vi "SubMatrix.vi"() -> ()   [LabVIEW 2014]
uses:
  <vilib>/Utility/file.llb/Read From Spreadsheet File (I64).vi
panel:
  in  "From V2 to 0":bool caption="From 0 to V1"
  in  "GPIB":string="12"
  in  "Sweep Rate w/o recording (V/min)":dbl=30.0
  in  "From V1 to V2":bool=TRUE
  in  "From 0 to V1":bool
  in  "Sweep Rate (V/min)":dbl=0.6
  in  "Menu Ring":u16(ring) caption="Show configuration:" items=["Configuration #1", "Configuration #2", "Configuration #3"]
  in  "Start Sweep":bool
  out "# of configurations":dbl
  out "Configuration file:":path
  in  "V2 (V)":dbl=2.1
  in  "V1 (V)":dbl=-2.1
  out "Array":bool[][](array[boolean])
  # "Which part of sweep to be recorded?"
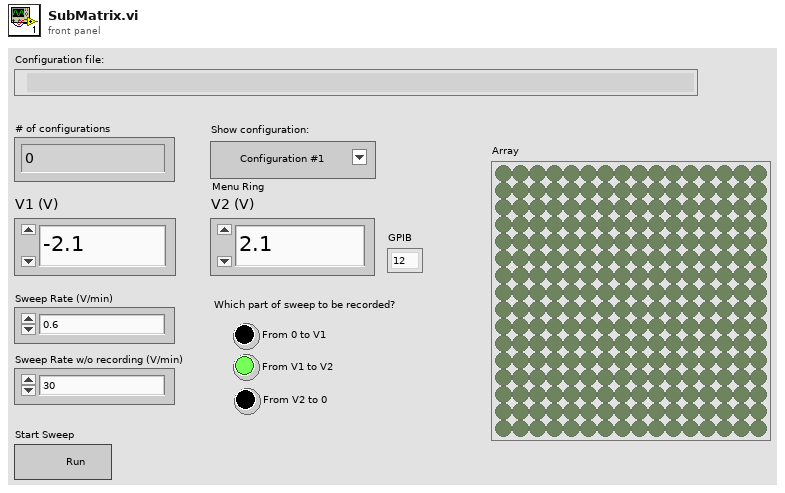
[diagram p1: front panel]
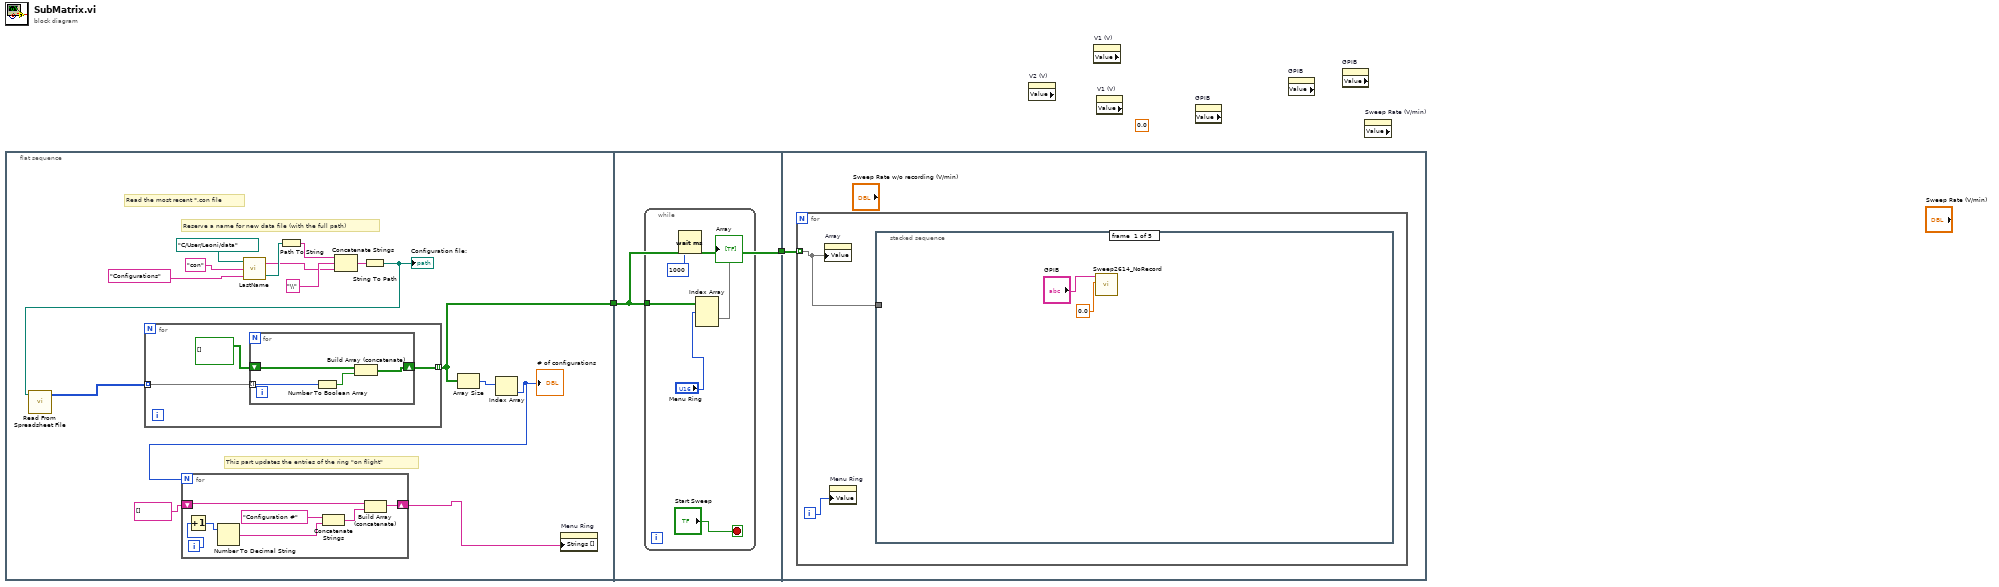
[diagram p0: block diagram]
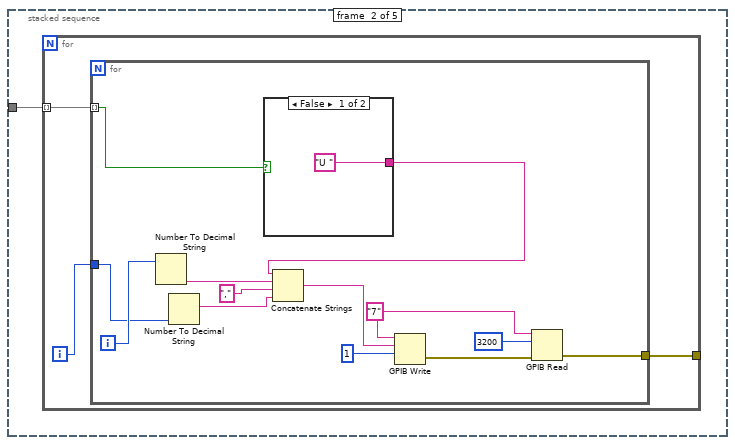
[diagram p2: hidden frame]
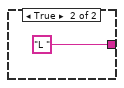
[diagram p3: hidden frame]
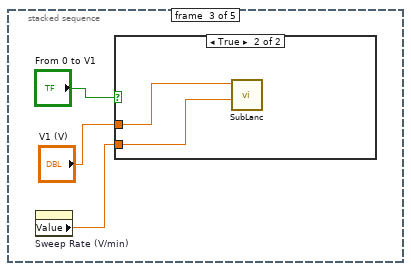
[diagram p4: hidden frame]
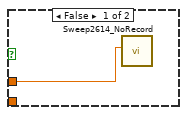
[diagram p5: hidden frame]
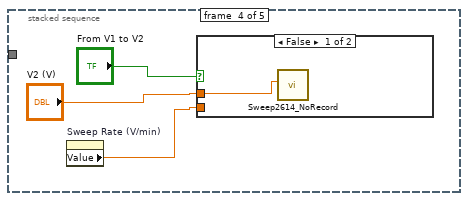
[diagram p6: hidden frame]
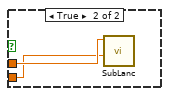
[diagram p7: hidden frame]
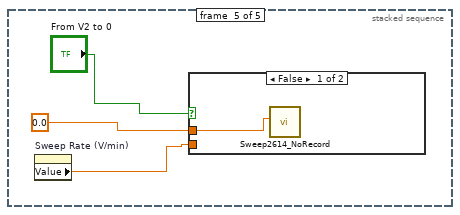
[diagram p8: hidden frame]
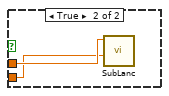
[diagram p9: hidden frame]
diagram:
  (unwired) 0.0
  n1 = flat-sequence {
    tunnel: [w4] -> w2
    tunnel: w2 -> [w32]
    tunnel: [w32] -> w1
    tunnel: w1 -> [w38]
    frame #0 {
      # "This part updates the entries of the ring \"on flight\""
      # "Reserve a name for new data file (with the full path)"
      # "Read the most recent *.con file"
      n2 = call "LastName.vi"("Custom Folder"="Configurations", "Extention"="con", "User Data Folder"=path "C:/User/Leoni/data") -> ("created path"=w13:path, "String"=w12:string)
      n3 = Path To String(path=w13) -> (string=w17:string)
      n4 = Concatenate Strings(w17, "\\", w12) -> (w15:string)
      n5 = String To Path(string=w15) -> (path=w9:path)
      "Configuration file:" <- w9
      n6 = call-poly <vilib>:"Read From Spreadsheet File.vi"("file path (dialog if empty)"=w9) -> ("all rows"=w8:i64[][])  [unwired: 6 in, 4 out]
      n7 = for {
        tunnel: w8 -> [w27] mode=indexing
        tunnel: [w26] -> w4 mode=indexing
        n8 = for {
          tunnel: w27 -> [w31] mode=indexing
          shift-right: [w28] -> w26
          shift-left: bool[][] [] -> [w29]
          n9 = Number To Boolean Array(number=w31) -> (Boolean array=w30:bool[])
          n10 = Build Array (concatenate)(w29, w30) -> (w28:bool[][])
        }
      }
      n11 = Array Size(array=w4) -> (size(s)=w7:i32[])
      n12 = Index Array(array=w7) -> (element=w5:i32)  [unwired: 1 in]
      "# of configurations" <- w5
      n13 = for {
        N: w5 -> [_]
        shift-right: [w21] -> w3
        shift-left: string[] [] -> [w22]
        i -> [w19]
        n14 = Increment(x=w19) -> (x+1=w18:i32)
        n15 = Number To Decimal String(number=w18) -> (decimal integer string=w23:string)  [unwired: 1 in]
        n16 = Concatenate Strings("Configuration #", w23) -> (w20:string)
        n17 = Build Array (concatenate)(w22, w20) -> (w21:string[])
      }
      n18 = property on="Menu Ring" class="Ring (strict)"("Strings []"=w3) -> ()  [unwired: 2 in, 2 out]
    }
    frame #1 {
      n19 = while {
        tunnel: w32 -> [w37]
        stop <- "Start Sweep" stop-if-true
        n20 = Wait (ms)(milliseconds to wait=1000) -> ()  [unwired: 1 out]
        n21 = Index Array(array=w37, index (dim 0)="Menu Ring") -> (element=→"Array":bool[][])  [unwired: 2 in]
      }
    }
    frame #2 {
      n22 = for {
        tunnel: w38 -> [w39] mode=indexing
        i -> [w40]
        n23 = property on="Array" class="Arr (strict)"("Value"=w39) -> ()  [unwired: 2 in, 2 out]
        n24 = property on="Menu Ring" class="Ring (strict)"("Value"=w40) -> ()  [unwired: 2 in, 2 out]
        n25 = stacked-sequence {
          tunnel: w39 -> [_ w43 _ _ _]
          frame #0 {
            n26 = call "Sweep2614_NoRecord.vi"("Vfinal (V)"=0.0, "GPIB"="GPIB") -> ()  [unwired: 2 in, 1 out]
          }
          frame #1 {
            n27 = for {
              tunnel: [w45] -> _
              tunnel: w43 -> [w44] mode=indexing
              i -> [w46]
              n28 = for {
                tunnel: w46 -> [w48]
                tunnel: [w51] -> w45
                tunnel: w44 -> [w47] mode=indexing
                i -> [w49]
                w53 = "7"
                n29 = Number To Decimal String(number=w49) -> (decimal integer string=w58:string)  [unwired: 1 in]
                n30 = Number To Decimal String(number=w48) -> (decimal integer string=w57:string)  [unwired: 1 in]
                n31 = case shown="False" w47 {
                  tunnel: ["U " "L "] -> w59
                  frame False {
                  }
                  frame True {
                  }
                }
                n32 = Concatenate Strings(w59, w58, ",", w57) -> (w50:string)
                n33 = GPIB Write(0:w53, 1:w50, 2:1) -> (6:w55:errorcluster)  [unwired: 2 in, 1 out]
                n34 = GPIB Read(0:w53, 1:3200, 3:w55) -> (7:w51:errorcluster)  [unwired: 2 in, 2 out]
              }
            }
          }
          frame #2 {
            n35 = property on="Sweep Rate (V/min)" class="DigNum (strict)"() -> ("Value"=w62:dbl)  [unwired: 2 in, 2 out]
            n36 = case shown="True" "From 0 to V1" {
              tunnel: "V1 (V)" -> [w65 w67]
              tunnel: w62 -> [_ w66]
              frame False {
                n37 = call "Sweep2614_NoRecord.vi"("Vfinal (V)"=w65) -> ()  [unwired: 3 in, 1 out]
              }
              frame True {
                n38 = call "SubLanc.vi"("Target Voltage, V"=w67, "Sweep rate, V/min"=w66) -> ()  [unwired: 8 in]
              }
            }
          }
          frame #3 {
            n39 = property on="Sweep Rate (V/min)" class="DigNum (strict)"() -> ("Value"=w68:dbl)  [unwired: 2 in, 2 out]
            n40 = case shown="False" "From V1 to V2" {
              tunnel: "V2 (V)" -> [w71 w73]
              tunnel: w68 -> [_ w72]
              frame False {
                n41 = call "Sweep2614_NoRecord.vi"("Vfinal (V)"=w71) -> ()  [unwired: 3 in, 1 out]
              }
              frame True {
                n42 = call "SubLanc.vi"("Target Voltage, V"=w73, "Sweep rate, V/min"=w72) -> ()  [unwired: 8 in]
              }
            }
          }
          frame #4 {
            n43 = property on="Sweep Rate (V/min)" class="DigNum (strict)"() -> ("Value"=w76:dbl)  [unwired: 2 in, 2 out]
            n44 = case shown="False" "From V2 to 0" {
              tunnel: 0.0 -> [w77 w79]
              tunnel: w76 -> [_ w78]
              frame False {
                n45 = call "Sweep2614_NoRecord.vi"("Vfinal (V)"=w77) -> ()  [unwired: 3 in, 1 out]
              }
              frame True {
                n46 = call "SubLanc.vi"("Target Voltage, V"=w79, "Sweep rate, V/min"=w78) -> ()  [unwired: 8 in]
              }
            }
          }
        }
      }
    }
  }
  n47 = property on="V2 (V)" class="DigNum (strict)" props=["Value"]() -> ()  [unwired: 2 in, 3 out]
  n48 = property on="V1 (V)" class="DigNum (strict)" props=["Value"]() -> ()  [unwired: 2 in, 3 out]
  n49 = property on="V1 (V)" class="DigNum (strict)" props=["Value"]() -> ()  [unwired: 2 in, 3 out]
  n50 = property on="GPIB" class="Str" props=["Value"]() -> ()  [unwired: 2 in, 3 out]
  n51 = property on="GPIB" class="Str" props=["Value"]() -> ()  [unwired: 2 in, 3 out]
  n52 = property on="GPIB" class="Str" props=["Value"]() -> ()  [unwired: 2 in, 3 out]
  n53 = property on="Sweep Rate (V/min)" class="DigNum (strict)" props=["Value"]() -> ()  [unwired: 2 in, 3 out]
